vi "test_MonoOpenAndInit.vi"(6 "Delay between send and receive [ms]":i32=100, 7 "Test should pass":bool=TRUE, 8 "error in":errorcluster, 9 "tear down connection":bool=TRUE, 10 "set-up a connection":bool=TRUE, 11 "device selection":enum16{"monochromator", "CCD", "SCD"}(ring)) -> (0 "error out":errorcluster, 1 "log-file path":path)   [LabVIEW 2023, in "horiba.test.lvlib"]
uses:
  Classes/Mono/Monochromator.lvclass
  <vilib>/addons/_JKI Toolkits/Caraya/classes/Assert/Assert Equal Value and Type_Variant.vi
  <vilib>/addons/_JKI Toolkits/Caraya/classes/Assert/Assert Not Error.vi
  horiba.test.lvlib
  <vilib>/addons/_JKI Toolkits/Caraya/classes/Test/Test.lvclass
  <vilib>/addons/_JKI Toolkits/Caraya/classes/Assert/Assert.lvclass
  Classes/horiba.lvlib
  <vilib>/Hampel Software Engineering/HSE Logger/hse-logger.lvlib
  C:/Projects/Horiba/horiba-labview-sdk/Source/Classes/GenericDevice/GenericDevice.lvclass
  C:/Projects/Horiba/horiba-labview-sdk/Source/Classes/Mono/Monochromator.lvclass
panel:
  in  "total time out [minutes]":i32=3
  # "Connector Pane"
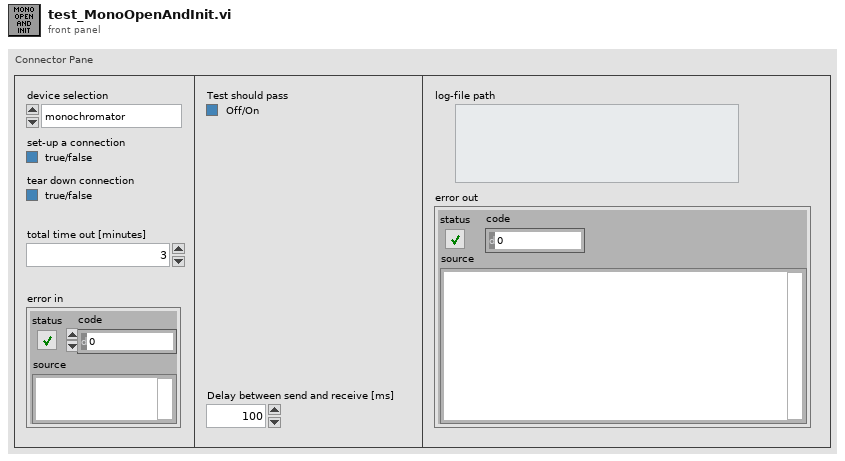
[diagram p1: front panel]
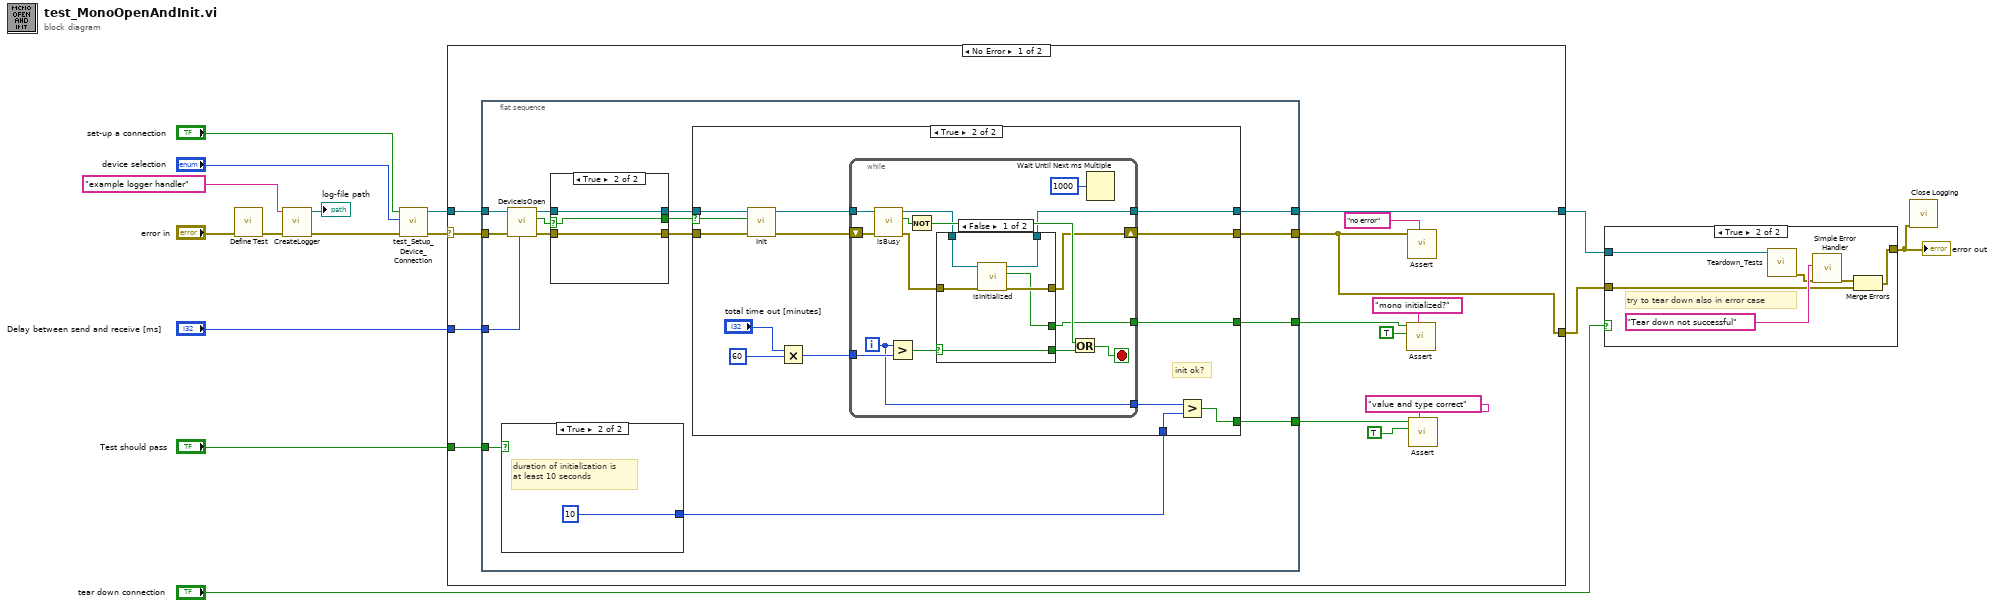
[diagram p0: block diagram]
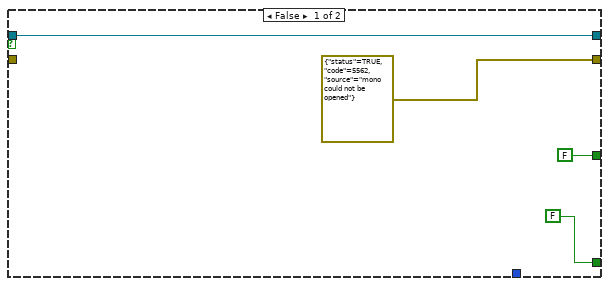
[diagram p2: hidden frame]
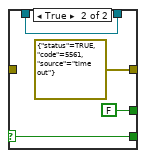
[diagram p3: hidden frame]
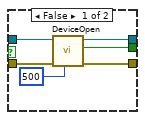
[diagram p4: hidden frame]
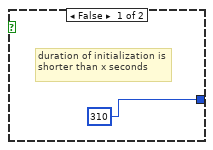
[diagram p5: hidden frame]
diagram:
  n1 = call <vilib>:"Define Test.vi"("error in (no error)"="error in") -> ("error out"=w6:errorcluster)  [unwired: 9 in, 1 out]
  n2 = call "CreateLogger.vi"("error in (no error)"=w6, "Handler Name"="example logger handler") -> ("error out"=w4:errorcluster, "log-file path"=→"log-file path":path)  [unwired: 8 in]
  n3 = call "test_Setup_Device_Connection.vi"("error in (no error)"=w4, "device selection"="device selection", "set-up a connection"="set-up a connection") -> ("error out"=w7:errorcluster, "Monochromator out"=w10:refnum<class "Monochromator.lvclass">)  [unwired: 5 in, 2 out]
  n4 = case shown="No Error" w7 {
    selector: w7 -> [w23 w99]
    tunnel: "Test should pass" -> [w26 _]
    tunnel: [w25 w98] -> w11
    tunnel: w10 -> [w24 w98]
    tunnel: [w16 w99] -> w8
    tunnel: "Delay between send and receive [ms]" -> [w22 _]
    frame No Error {
      n5 = flat-sequence {
        tunnel: w23 -> [w42]
        tunnel: w26 -> [w43]
        tunnel: [w32] -> w25
        tunnel: w24 -> [w39]
        tunnel: w22 -> [w38]
        tunnel: [w31] -> w21
        tunnel: [w30] -> w16
        tunnel: [w29] -> w17
        frame #0 {
          n6 = case shown="True" w43 {
            tunnel: [310 ("y") 10 ("y")] -> w33
            frame False {
              # "duration of initialization is shorter than x seconds"
            }
            frame True {
              # "duration of initialization is at least 10 seconds"
            }
          }
          n7 = call-dynamic "DeviceIsOpen.vi"("Delay between send and receive [ms]"=w38, "error in (no error)"=w42, "Monochromator in"=w39) -> ("error out"=w40:errorcluster, "device is open?"=w37:bool, "Monochromator out"=w41:refnum<class "Monochromator.lvclass">)  [unwired: 5 in, 1 out]
          n8 = case shown="True" w37 {
            selector: w37 -> [_ w93]
            tunnel: w41 -> [w92 w95]
            tunnel: [w89 w95] -> w34
            tunnel: w40 -> [w91 w94]
            tunnel: [w90 w94] -> w35
            tunnel: [w87 w93] -> w36
            frame False {
              n9 = call-dynamic "DeviceOpen.vi"("Delay between send and receive [ms]"=500, "error in (no error)"=w91, "Monochromator in"=w92) -> ("error out"=w90:errorcluster, "device is open?"=w87:bool, "Monochromator out"=w89:refnum<class "Monochromator.lvclass">)  [unwired: 5 in, 1 out]
            }
            frame True {
            }
          }
          n10 = case shown="True" w36 {
            selector: w36 -> [_ w60]
            tunnel: w35 -> [_ w59]
            tunnel: w34 -> [w45 w61]
            tunnel: [errorcluster {"status"=TRUE, "code"=5562, "source"="mono could not be opened"} ("error in 2") w52] -> w30
            tunnel: [FALSE w51] -> w31
            tunnel: w33 -> [_ w50]
            tunnel: [w45 w49] -> w32
            tunnel: [FALSE w48] -> w29
            frame False {
            }
            frame True {
              # "init ok?"
              n11 = call "Init.vi"("error in (no error)"=w59, "force"=w60, "Monochromator in"=w61) -> ("error out"=w57:errorcluster, "Monochromator out"=w58:refnum<class "Monochromator.lvclass">)  [unwired: 5 in, 2 out]
              n12 = Multiply(x="total time out [minutes]", y=60) -> (x*y=w54:i32)
              n13 = while {
                tunnel: w58 -> [w76]
                tunnel: w54 -> [w71]
                shift-right: [w66] -> w52
                shift-left: w57 -> [w75]
                tunnel: [w65] -> w53
                tunnel: [w63] -> w49
                tunnel: [w62] -> w48
                i -> [w65]
                stop <- w70 stop-if-true
                n14 = call "isBusy.vi"("error in (no error)"=w75, "Monochromator in"=w76) -> ("error out"=w67:errorcluster, "mono is busy?"=w72:bool, "Monochromator out"=w64:refnum<class "Monochromator.lvclass">)  [unwired: 7 in]
                n15 = Greater?(x=w65, y=w71) -> (0:w69:bool)
                n16 = Not(x=w72) -> (.not. x?=w73:bool)
                n17 = case shown="False" w69 {
                  selector: w69 -> [w82 w86]
                  tunnel: [w82 w86] -> w68
                  tunnel: w67 -> [w80 _]
                  tunnel: [w81 errorcluster {"status"=TRUE, "code"=5561, "source"="time out"} ("error in 2")] -> w66
                  tunnel: w64 -> [w79 w84]
                  tunnel: [w78 w84] -> w63
                  tunnel: [w77 FALSE] -> w62
                  frame False {
                    n18 = call "isInitialized.vi"("error in (no error)"=w80, "Monochromator in"=w79) -> ("error out"=w81:errorcluster, "mono is initialized?"=w77:bool, "Monochromator out"=w78:refnum<class "Monochromator.lvclass">)  [unwired: 7 in]
                  }
                  frame True {
                  }
                }
                n19 = Or(x=w73, y=w68) -> (x .or. y?=w70:bool)
                n20 = Wait Until Next ms Multiple(millisecond multiple=u32 1000) -> ()  [unwired: 1 out]
              }
              n21 = Greater?(x=w53, y=w50) -> (0:w51:bool)
            }
          }
        }
      }
      n22 = call-poly <vilib>:"Assert.vi"("Label"="mono initialized?" ("Label (VI Title)"), "Y"=TRUE, "X"=w17) -> ()  [unwired: 7 in, 2 out]
      n23 = call-poly <vilib>:"Assert.vi"("Label"="no error" ("Label (VI Title)"), "Not Error?"=w16) -> ()  [unwired: 8 in, 2 out]
      n24 = call-poly <vilib>:"Assert.vi"("Label"="value and type correct" ("Label (VI Title)"), "Y"=TRUE, "X"=w21) -> ()  [unwired: 7 in, 2 out]
    }
    frame Error {
    }
  }
  n25 = case shown="True" "tear down connection" {
    tunnel: w11 -> [_ w105]
    tunnel: [w100 w101] -> w2
    tunnel: w8 -> [w100 w102]
    frame False {
    }
    frame True {
      # "try to tear down also in error case"
      n26 = call "Teardown_Tests.vi"("horiba.lvlib:GenericDevice"=w105) -> ("error out"=w104:errorcluster)  [unwired: 9 in, 1 out]
      n27 = call <vilib>:"Simple Error Handler.vi"("error source (\" \")"="Tear down not successful" ("error source (\" \")"), "error in (no error)"=w104) -> ("error out"=w103:errorcluster)  [unwired: 3 in, 4 out]
      n28 = Merge Errors(w103, w102) -> (w101:errorcluster)
    }
  }
  "error out" <- w2
  n29 = call <vilib>:"Close Logging.vi"("error in"=w2) -> ()  [unwired: 10 in, 1 out]
